vi "Digital Read Multiple Channels.vi"(8 "error in (no error)":errorcluster, 10 "Array":i32[](array[numeric]), 11 "NI-DAQ in":refnum<class "NI-DAQ.lvclass">) -> (0 "error out":errorcluster, 2 "subarray":bool[](array[boolean]), 3 "NI-DAQ out":refnum<class "NI-DAQ.lvclass">)   [LabVIEW 2019, in "NI-DAQ.lvclass"]
uses:
  NI-DAQ.lvclass
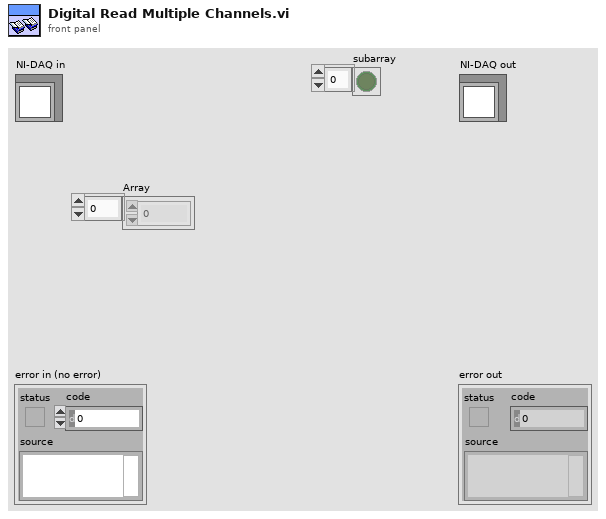
[diagram p1: front panel]
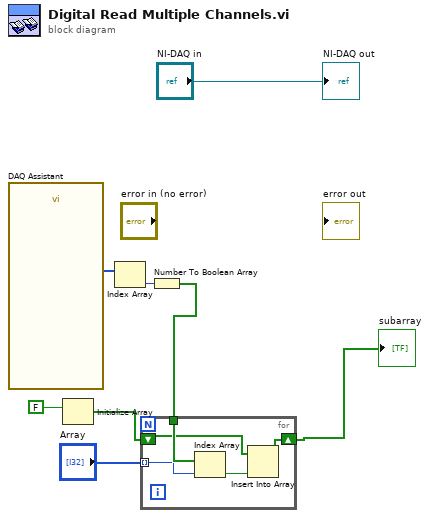
[diagram p0: block diagram]
diagram:
  n1 = call "DAQ Assistant"() -> ("data"=w7:u32[])  [unwired: 17 in, 2 out]
  n2 = Initialize Array(FALSE) -> (w2:bool[])  [unwired: 1 in]
  n3 = Index Array(array=w7) -> (element=w8:u32)  [unwired: 1 in]
  n4 = Number To Boolean Array(number=w8) -> (Boolean array=w5:bool[])
  n5 = for {
    tunnel: w5 -> [w13]
    tunnel: "Array" -> [w12] mode=indexing
    shift-right: [w11] -> w3
    shift-left: w2 -> [w10]
    n6 = Index Array(array=w13, index=w12) -> (element=w9:bool)
    n7 = Insert Into Array(array=w10, new element=w9) -> (w11:bool[])  [unwired: 1 in]
  }
  "subarray" <- w3
  "NI-DAQ out" <- "NI-DAQ in"
